vi "Pcre2SubstringNumberFromName8.vi"(8 "error in":errorcluster, 10 "Name":string, 11 "pCode":u64 format="%.0x") -> (0 "error out":errorcluster, 2 "Number":i32, 3 "pCode":u64 format="%.0x")   [LabVIEW 2021, in "libpcre2-8.lvlib"]
uses:
  libpcre2-8.lvlib
  libpcre2-8-x32.dll
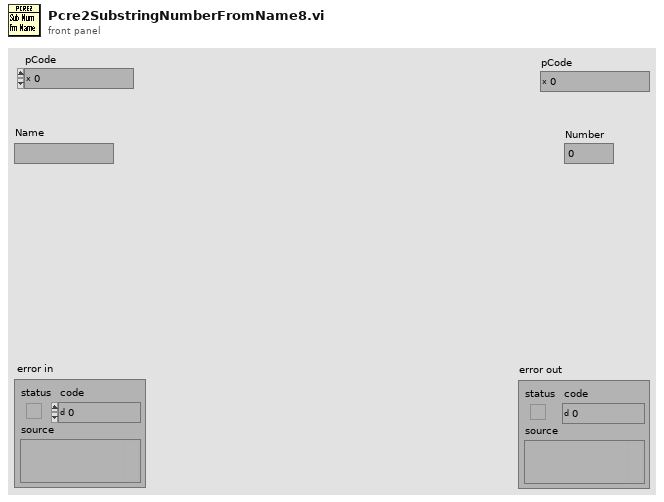
[diagram p1: front panel]
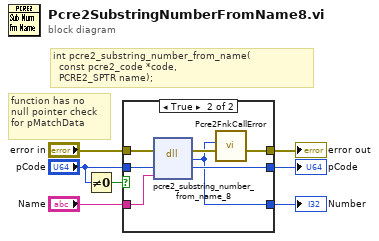
[diagram p0: block diagram]
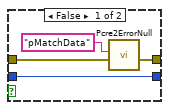
[diagram p2: hidden frame]
diagram:
  # "function has no \nnull pointer check \nfor pMatchData"
  # "int pcre2_substring_number_from_name(\n  const pcre2_code *code,\n  PCRE2_SPTR name);"
  n1 = Not Equal To 0?(x="pCode") -> (x != 0?=w4:bool)
  n2 = case shown="True" w4 {
    tunnel: "error in" -> [w10 w18]
    tunnel: [w9 w14] -> w6
    tunnel: "pCode" -> [w11 w17]
    tunnel: [w11 w16] -> w5
    tunnel: "Name" -> [_ w13]
    tunnel: [_ w12] -> w1
    frame False {
      n3 = call "Pcre2ErrorNull.vi"("error in"=w10, "What"="pMatchData" ("message")) -> ("error out"=w9:errorcluster)  [unwired: 9 in]
    }
    frame True {
      n4 = dll-call lib="libpcre2-8-x*.dll" fn="pcre2_substring_number_from_name_8"(error in=w18, "code"=w17, "number"=w13) -> (error out=w15:errorcluster, "number"=w12:i32, "code"=w16:u64)  [unwired: 3 in, 1 out]
      n5 = call "Pcre2FnkCallError.vi"("error in"=w15, "ErrorCode"=w12) -> ("error out"=w14:errorcluster)  [unwired: 9 in]
    }
  }
  "pCode" <- w5
  "error out" <- w6
  "Number" <- w1
